vi "GetAvailableSensitivities.vi"(8 "error in (no error)":errorcluster, 11 "dSensitivities":dbl) -> (0 "error out":errorcluster, 2 "function return":i16, 3 "dSensitivities out":dbl)   [LabVIEW 2013, in "HS3OverallRoutines.lvlib"]
doc: "This routine retrieves the available input sensitivities from the\nhardware and stores them in an array. dSensitivities is a 20 elements large array. The caller must ensure that there is enough space in the array to contain the data. Therefore the size of the array in bytes must be at least 20 * sizeof(double) At return, all elements containing a non-zero value, contain an input sensitivity. This is a full scale value. So if an element contains the value 4.0, the input sensitivity is 4 Volt full scale, enabling to measure input signals from -4 Volt - +4 Volt.\n\ninput: -\noutput: dSensitivities the array of input sensitivities\nReturn value E_NO_ERRORS | E_NO_HARDWARE\n\nFunction prototype: word GetAvailableSensitivities( double *dSensitivities )\n\nshort int GetAvailableSensitivities ( double *dSensitivities );"
uses:
  HS3OverallRoutines.lvlib
  hs3.dll
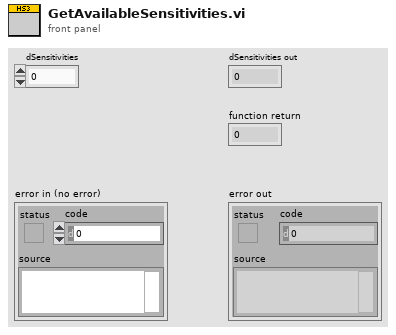
[diagram p1: front panel]
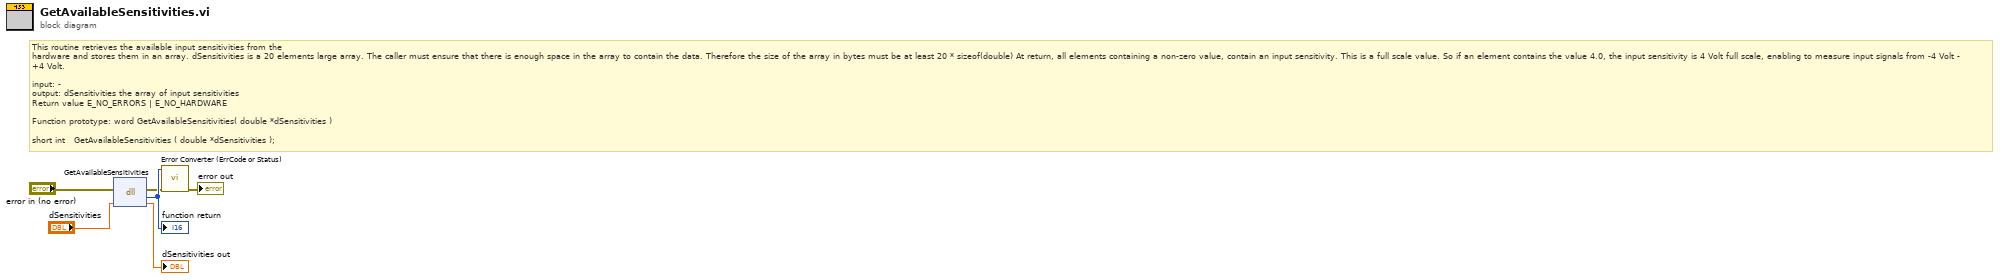
[diagram p0: block diagram]
diagram:
  # "This routine retrieves the available input sensitivities from the\nhardware and stores them in an array. dSensitivities is a 20 elements large array. The caller must ensure that there is enough space in the array to contain the data. Therefore the size of the array in bytes must be at least 20 * sizeof(double) At return, all elements containing a non-zero value, contain an input sensitivity. This is a full scale value. So if an element contains the value 4.0, the input sensitivity is 4 Volt full scale, enabling to measure input signals from -4 Volt - +4 Volt.\n\ninput: -\noutput: dSensitivities the array of input sensitivities\nReturn value E_NO_ERRORS | E_NO_HARDWARE\n\nFunction prototype: word GetAvailableSensitivities( double *dSensitivities )\n\nshort int \t\tGetAvailableSensitivities\t( double *dSensitivities );"
  n1 = dll-call lib="C:/Documents and Settings/admin/Pulpit/HS3 LabViewLib/HS3_WRAPPER/OverallRoutines/hs3.*" fn="GetAvailableSensitivities"(error in="error in (no error)", "dSensitivities"="dSensitivities") -> (error out=w2:errorcluster, w6:i16, "dSensitivities"=→"dSensitivities out":dbl)  [unwired: 2 in, 1 out]
  "function return" <- w6
  n2 = call "Error Converter (ErrCode or Status).vi"("error in (no error)"=w2, "error code"=w6) -> ("error out"=→"error out":errorcluster)  [unwired: 9 in]
